vi "Read Actuator.vi"(11 "Model in":refnum<class "Model.lvclass">) -> (2 "IActuator.lvclass":refnum<class "IActuator.lvclass">, 3 "Model out":refnum<class "Model.lvclass">)   [LabVIEW 2015, in "Model.lvclass"]
uses:
  Model.lvclass
  Actuator/IActuator/IActuator.lvclass
  Model.lvclass/Model.ctl
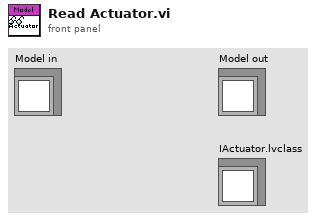
[diagram p1: front panel]
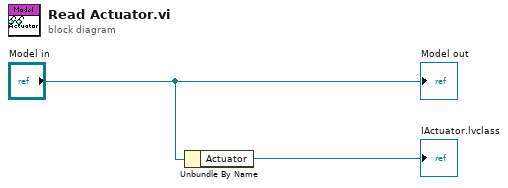
[diagram p0: block diagram]
diagram:
  n1 = Unbundle By Name("Model in") -> ("Actuator"=→"IActuator.lvclass":refnum<class "IActuator.lvclass">)
  "Model out" <- "Model in"
